vi "loadRampDetails.vi"(8 "error in (no error)":errorcluster, 10 "RampEvent in":refnum<class "RampEvent.lvclass">, 11 "RampAction in":refnum<class "RampAction.lvclass">) -> (0 "error out":errorcluster, 2 "RampEvent out":refnum<class "RampEvent.lvclass">, 3 "RampAction out":refnum<class "RampAction.lvclass">)   [LabVIEW 2011, in "Views.lvlib" / "ScriptEditor.lvlib" / "RampAction.lvclass"]
uses:
  RampAction.lvclass
  Tools/Scripting/ScriptingEvent/ScriptEvents/Ramp/RampEvent/RampEvent.lvclass
  RampAction.lvclass/RampAction.ctl
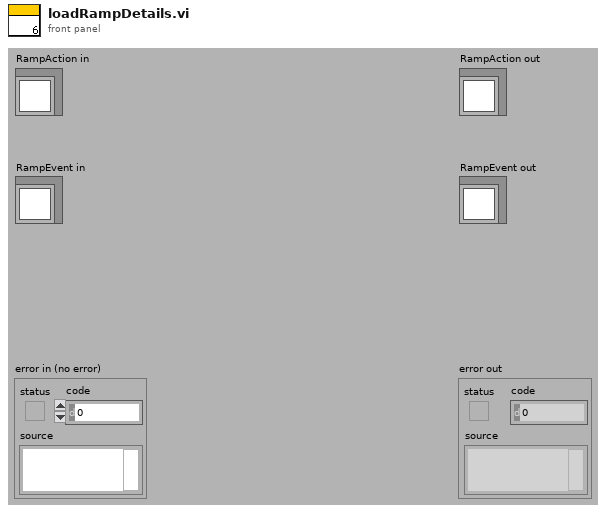
[diagram p1: front panel]
types:
  T1 = cluster{"rampTime":dbl, "timeStep":dbl, "dataValueStep":dbl}
  T2 = typedef "LVStringsAndValuesArrayTypeDef.ctl" = cluster{"String":string, "Value":u16}[]
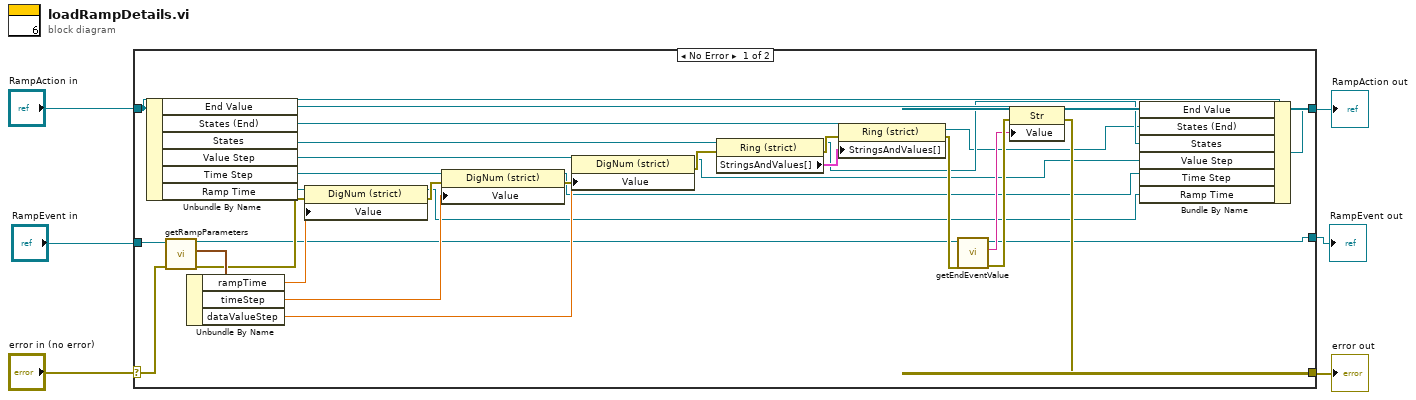
[diagram p0: block diagram]
diagram:
  n1 = case shown="No Error" "error in (no error)" {
    selector: "error in (no error)" -> [w37 w40]
    tunnel: [w16 w40] -> w5
    tunnel: [w8 w39] -> w3
    tunnel: "RampAction in" -> [w15 w39]
    tunnel: "RampEvent in" -> [w38 _]
    tunnel: [w7 _] -> w1
    frame No Error {
      n2 = Unbundle By Name(w15) -> ("End Value"=w21:refnum<vi>, "States (End)"=w25:refnum<vi>, "States"=w26:refnum<vi>, "Value Step"=w28:refnum<vi>, "Time Step"=w32:refnum<vi>, "Ramp Time"=w35:refnum<vi>)
      n3 = call "getRampParameters.vi"("error in (no error)"=w37, "RampEvent in"=w38) -> ("error out"=w33:errorcluster, "RampParameters"=w36:T1, "RampEvent out"=w19:refnum<class "RampEvent.lvclass">)  [unwired: 7 in]
      n4 = Unbundle By Name(w36) -> ("rampTime"=w34:dbl, "timeStep"=w30:dbl, "dataValueStep"=w27:dbl)
      n5 = property class="DigNum (strict)"(reference=w35, error in=w33, "Value"=w34) -> (reference out=w14:refnum<vi>, error out=w31:errorcluster)
      n6 = property class="DigNum (strict)"(reference=w32, error in=w31, "Value"=w30) -> (reference out=w13:refnum<vi>, error out=w29:errorcluster)
      n7 = property class="DigNum (strict)"(reference=w28, error in=w29, "Value"=w27) -> (reference out=w12:refnum<vi>, error out=w24:errorcluster)
      n8 = property class="Ring (strict)"(reference=w26, error in=w24) -> (reference out=w11:refnum<vi>, error out=w23:errorcluster, "StringsAndValues[]"=w22:T2)
      n9 = property class="Ring (strict)"(reference=w25, error in=w23, "StringsAndValues[]"=w22) -> (reference out=w10:refnum<vi>, error out=w20:errorcluster)
      n10 = call "getEndEventValue.vi"("error in (no error)"=w20, "RampEvent in"=w19) -> ("error out"=w18:errorcluster, "newValue"=w17:string, "RampEvent out"=w7:refnum<class "RampEvent.lvclass">)  [unwired: 7 in]
      n11 = property class="Str"(reference=w21, error in=w18, "Value"=w17) -> (reference out=w9:refnum<vi>, error out=w16:errorcluster)
      n12 = Bundle By Name(cluster=w15, "End Value"=w9, "States (End)"=w10, "States"=w11, "Value Step"=w12, "Time Step"=w13, "Ramp Time"=w14) -> (w8:refnum<class "RampAction.lvclass">)
    }
    frame Error {
    }
  }
  "error out" <- w5
  "RampAction out" <- w3
  "RampEvent out" <- w1
